vi "VISA_RST.vi"(6 "UseOPC?(T)":bool, 8 "error in":errorcluster {"code" format="%.0x"}, 9 "Timeout":u32=3000, 11 "Session In":refnum<visa-resource-name>="GPIB0::4::INSTR") -> (0 "error out":errorcluster {"code" format="%.0x"}, 3 "Session Out":refnum<visa-resource-name>)   [LabVIEW 2018]
doc: "Launches the Instrument I/O Assistant, which you can use to communicate with message-based instruments and graphically parse the response. For example you can communicate with an instrument that uses a serial, Ethernet, or GPIB interface."
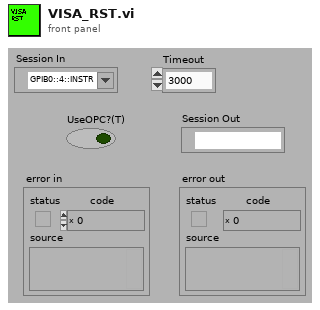
[diagram p1: front panel]
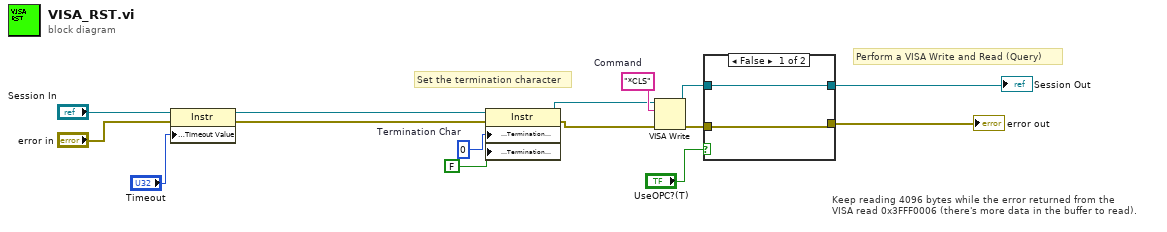
[diagram p0: block diagram]
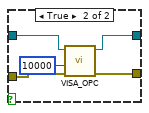
[diagram p2: hidden frame]
diagram:
  w7 = "*CLS"  # Command
  w9 = u8 0  # Termination Char
  # "Perform a VISA Write and Read (Query)"
  # "Keep reading 4096 bytes while the error returned from the\nVISA read 0x3FFF0006 (there's more data in the buffer to read)."
  # "Set the termination character"
  n1 = property class="Instr"(reference="Session In", error in="error in", "General Settings:Timeout Value"="Timeout") -> (reference out=w12:refnum<visa-resource-name>, error out=w11:errorcluster)
  n2 = property class="Instr"(reference=w12, error in=w11, "Message Based Settings:Termination Character"=w9, "Message Based Settings:Termination Character Enable"=FALSE ("enable")) -> (reference out=w5:refnum<visa-resource-name>, error out=w10:errorcluster)
  n3 = VISA Write(VISA resource name=w5, write buffer=w7, error in (no error)=w10) -> (VISA resource name out=w3:refnum<visa-resource-name>, error out=w6:errorcluster)  [unwired: 1 out]
  n4 = case shown="False" "UseOPC?(T)" {
    tunnel: w6 -> [w17 w22]
    tunnel: [w17 w21] -> w4
    tunnel: w3 -> [w16 w19]
    tunnel: [w16 w18] -> w2
    frame False {
    }
    frame True {
      n5 = call "VISA_OPC.vi"("error in"=w22, "Timeout"=u32 10000, "Session In"=w19) -> ("error out"=w21:errorcluster, "Session Out"=w18:refnum<visa-resource-name>)  [unwired: 6 in, 1 out]
    }
  }
  "error out" <- w4
  "Session Out" <- w2
